vi "Calculate Scaling Factor.vi"(10 "desired size":T1={"Horizontal"=-1, "Vertical"=-1}, 11 "unscaled size":T1={"Horizontal"=-1, "Vertical"=-1}) -> (3 "scaling factor":T2={"horizontal"=1.0, "vertical"=1.0} {"vertical" min=0.0; "horizontal" min=0.0})   [LabVIEW 2010, in "NI_SE_Front Panel Layout.lvlib"]
uses:
  NI_SE_Front Panel Layout.lvlib
  <vilib>/Utility/miscctls.llb/LVPointTypeDef.ctl
  XY Scaling Factor.ctl
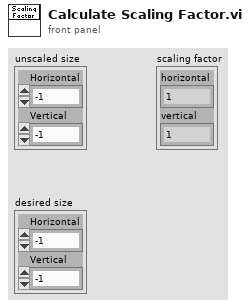
[diagram p1: front panel]
types:
  T1 = typedef "LVPointTypeDef.ctl" = cluster{"Horizontal":i16, "Vertical":i16}
  T2 = typedef "NI_SE_Front Panel Layout.lvlib/XY Scaling Factor.ctl" = cluster{"horizontal":dbl, "vertical":dbl}
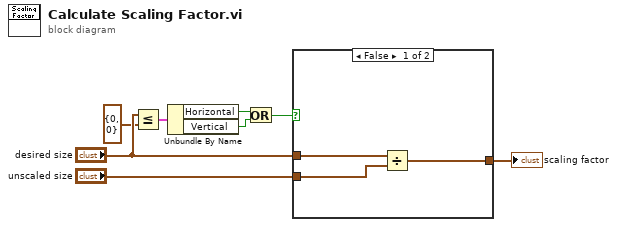
[diagram p0: block diagram]
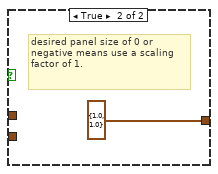
[diagram p2: hidden frame]
diagram:
  n1 = Less Or Equal?(x="desired size", y=T1 {"Horizontal"=0, "Vertical"=0}) -> (x <= y?=w5:cluster{"Horizontal":bool, "Vertical":bool})
  n2 = Unbundle By Name(w5) -> ("Horizontal"=w4:bool, "Vertical"=w3:bool)
  n3 = Or(x=w4, y=w3) -> (x .or. y?=w2:bool)
  n4 = case shown="False" w2 {
    tunnel: [w10 T2 {"horizontal"=1.0, "vertical"=1.0} ("scaling factor")] -> w8
    tunnel: "desired size" -> [w11 _]
    tunnel: "unscaled size" -> [w9 _]
    frame False {
      n5 = Divide(x=w11, y=w9) -> (x/y=w10:cluster{"Horizontal":dbl, "Vertical":dbl})
    }
    frame True {
      # "desired panel size of 0 or negative means use a scaling factor of 1."
    }
  }
  "scaling factor" <- w8
